vi "Punto 5.vi"() -> ()   [LabVIEW 2020]
panel:
  in  "Cancel Button":bool
  out "Second sorted array":dbl[](array[numeric])
  out "First sorted array":dbl[](array[numeric])
  in  "Original array":dbl[](array[numeric])
  # "This program was created by Juan Bermúdez from the Army Aviation School\nat the Aircraft Engineering of the assignature of Programation II"
  # "How to use the software?:\n1- First, write the numbers.\n2- Second, if you want to stop the software, push the buttom called = ''Cancel buttom''.\n Enjoy the software :)"
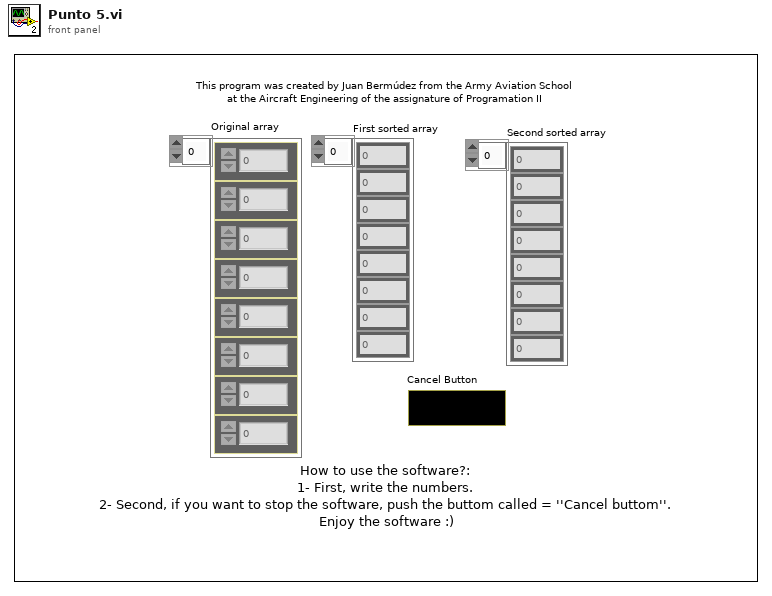
[diagram p1: front panel]
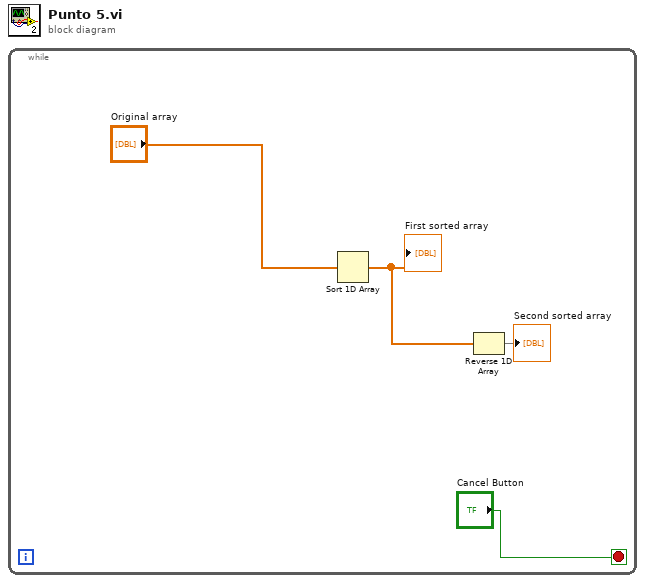
[diagram p0: block diagram]
diagram:
  n1 = while {
    stop <- "Cancel Button" stop-if-true
    n2 = Sort 1D Array(array="Original array") -> (sorted array=w3:dbl[])
    "First sorted array" <- w3
    n3 = Reverse 1D Array(array=w3) -> (reversed array=→"Second sorted array":dbl[])
  }
